vi "LWXPS_PositionerCompensationFrequencyNotchsGet.vi"(0 "XPS Reference IN":refnum<k24>, 1 "Positioner Name":string, 5 "LabVIEW error IN":errorcluster) -> (7 "LabVIEW error OUT":errorcluster, 8 "XPS Reference OUT":refnum<k24>, 9 "XPS Error String":string, 10 "Returned error code":i32, 11 "Notch Gain 3":dbl, 12 "Notch Frequency 1":dbl, 13 "Notch Bandwidth 3":dbl, 14 "Notch Bandwidth 1":dbl, 15 "Notch Gain 1":dbl, 16 "Notch Frequency 2":dbl, 17 "Notch Bandwidth 2":dbl, 18 "Notch Gain 2":dbl, 19 "Notch Frequency 3":dbl)   [LabVIEW 2014]
uses:
  D:/XPSQ8_LabView_Library/Development/Source/Dll/Newport.XPS.CommandInterface.dll
  Dll/Newport.XPS.CommandInterface.dll
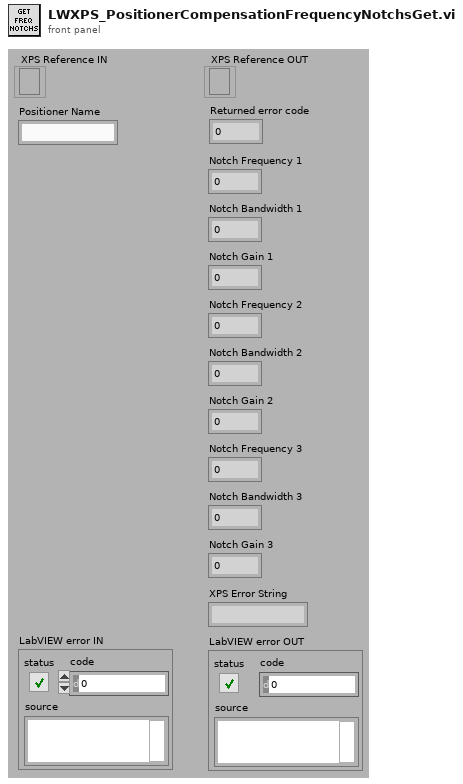
[diagram p1: front panel]
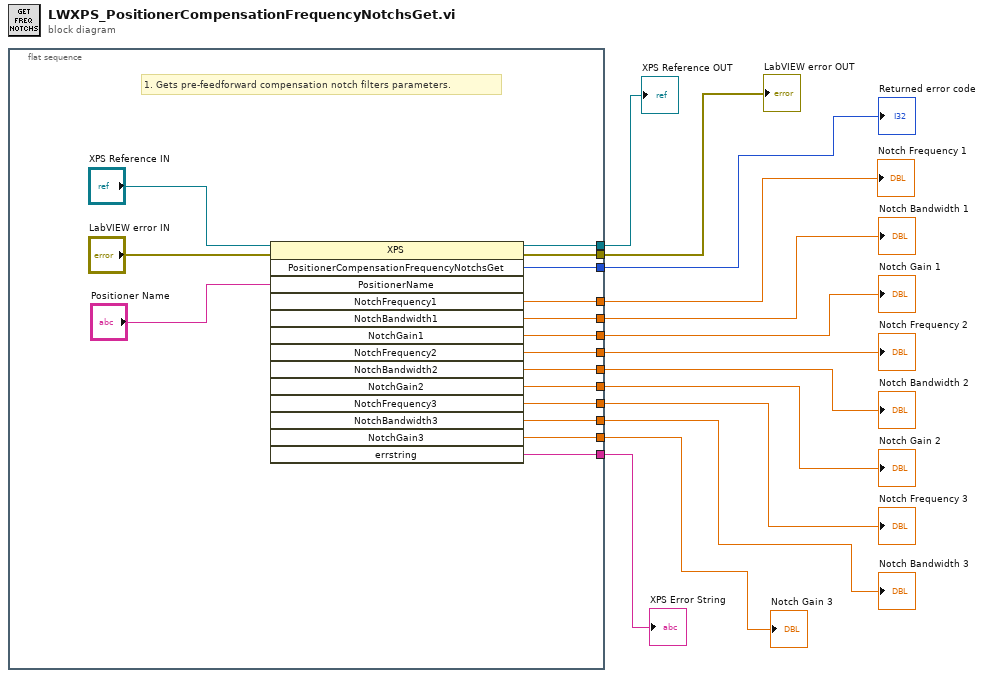
[diagram p0: block diagram]
diagram:
  n1 = flat-sequence {
    tunnel: [w26] -> w13
    tunnel: [w29] -> w12
    tunnel: [w28] -> w11
    tunnel: [w25] -> w5
    tunnel: [w24] -> w6
    tunnel: [w23] -> w7
    tunnel: [w22] -> w8
    tunnel: [w21] -> w1
    tunnel: [w20] -> w2
    tunnel: [w19] -> w10
    tunnel: [w18] -> w9
    tunnel: [w17] -> w3
    tunnel: [w16] -> w4
    frame #0 {
      # "1. Gets pre-feedforward compensation notch filters parameters."
      n2 = invoke class="XPS" method="PositionerCompensationFrequencyNotchsGet"(reference="XPS Reference IN", error in="LabVIEW error IN", "PositionerName"="Positioner Name") -> (reference out=w26:refnum<k24>, error out=w29:errorcluster, "PositionerCompensationFrequencyNotchsGet"=w28:i32, "NotchFrequency1"=w25:dbl, "NotchBandwidth1"=w24:dbl, "NotchGain1"=w23:dbl, "NotchFrequency2"=w22:dbl, "NotchBandwidth2"=w21:dbl, "NotchGain2"=w20:dbl, "NotchFrequency3"=w19:dbl, "NotchBandwidth3"=w18:dbl, "NotchGain3"=w17:dbl, "errstring"=w16:string)  [unwired: 11 in, 1 out]
    }
  }
  "XPS Reference OUT" <- w13
  "LabVIEW error OUT" <- w12
  "Returned error code" <- w11
  "XPS Error String" <- w4
  "Notch Gain 2" <- w2
  "Notch Frequency 3" <- w10
  "Notch Bandwidth 2" <- w1
  "Notch Bandwidth 3" <- w9
  "Notch Gain 3" <- w3
  "Notch Frequency 2" <- w8
  "Notch Gain 1" <- w7
  "Notch Bandwidth 1" <- w6
  "Notch Frequency 1" <- w5
